vi "Write groups.vi"(8 "error in (no error)":errorcluster, 10 "groups":string[](array[string]), 11 "[M] TDMS Save in":refnum<class "[M] TDMS Save.lvclass">) -> (0 "error out":errorcluster, 3 "[M] TDMS Save out":refnum<class "[M] TDMS Save.lvclass">)   [LabVIEW 2020, in "[M] TDMS Save.lvlib" / "[M] TDMS Save.lvclass"]
uses:
  [M] TDMS Save.lvclass
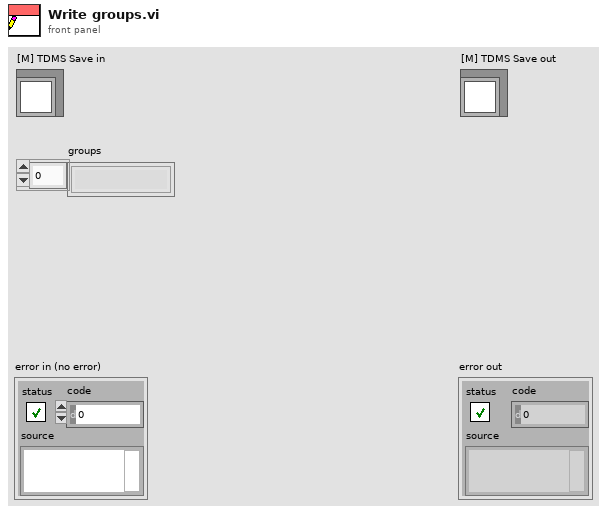
[diagram p1: front panel]
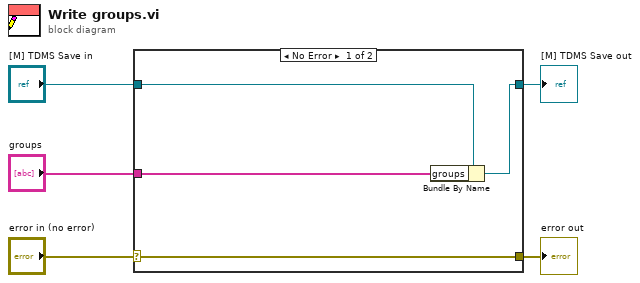
[diagram p0: block diagram]
diagram:
  n1 = case shown="No Error" "error in (no error)" {
    selector: "error in (no error)" -> [w9 w10]
    tunnel: [w9 w10] -> w4
    tunnel: [w7 w11] -> w2
    tunnel: "[M] TDMS Save in" -> [w8 w11]
    tunnel: "groups" -> [w6 _]
    frame No Error {
      n2 = Bundle By Name(cluster=w8, "groups"=w6) -> (w7:refnum<class "[M] TDMS Save.lvclass">)
    }
    frame Error {
    }
  }
  "error out" <- w4
  "[M] TDMS Save out" <- w2
